vi "Digital Read N Chans.vi"(8 "Error In":errorcluster, 10 "DI Channels":u8[](array[numeric]), 11 "LINX Resource":T1) -> (0 "Error Out":errorcluster, 2 "Values":bool[](array[boolean]), 3 "LINX Resource":T1)   [LabVIEW 2020, in "LMH-LINX.lvlib"]
doc: "Read the values of the specified digital input channels."
uses:
  LMH-LINX.lvlib
  Private/Type Defs/LINX Ref.ctl
  Private/Type Defs/Platform.ctl
  Private/Type Defs/Interface.ctl
  Private/Device/Type Defs/LINX Device Config.ctl
  Private/Device/Type Defs/TCP Config.ctl
  Private/Device/Type Defs/Channels.ctl
  Private/Type Defs/Peripheral.ctl
  Private/Utilties/Generate Error.vi
  Private/Device/Device.lvlib
  Private/Local IO/Local IO.lvlib
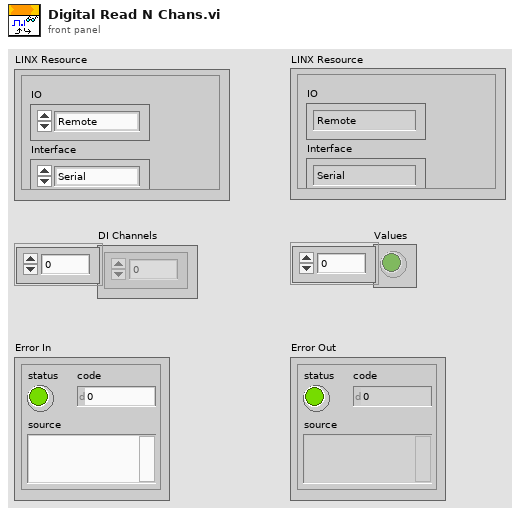
[diagram p1: front panel]
types:
  T1 = typedef "LMH-LINX.lvlib/LINX Ref.ctl" = cluster{"IO":T2, "Interface":T3, "LINX Device Config":T4}
  T2 = typedef "LMH-LINX.lvlib/Platform.ctl" = enum16{"Remote", "Local"}
  T3 = typedef "LMH-LINX.lvlib/Interface.ctl" = enum16{"Serial", "TCP"}
  T4 = typedef "LMH-LINX.lvlib/Device.lvlib/LINX Device Config.ctl" = cluster{"Interface":T3, "COM Port":refnum<visa-resource-name>, "TCP Configuration":T5, "Device Family":u8, "Device ID":u8, "Device Name":string, "TCP Ref":refnum<k5>, "Channels":T6}
  T5 = typedef "LMH-LINX.lvlib/Device.lvlib/TCP Config.ctl" = cluster{"IP Address":string, "Port":u16}
  T6 = typedef "LMH-LINX.lvlib/Channels.ctl" = cluster{"DI":u8[], "DO":u8[], "AI":u8[], "AO":u8[], "PWM":u8[], "QE":u8[], "UART":u8[], "I2C 2":u8[], "SPI":u8[], "CAN":u8[], "Servo":u8[], "AI Ref (V)":dbl, "AI Resolution (Bits)":u8, "AO Ref (V)":dbl, "AO Resolution (Bits)":u8}
  T7 = typedef "LMH-LINX.lvlib/Peripheral.ctl" = enum8{"DI", "DO", "AI", "AO", "PWM", "QE", "UART", "I2C", "SPI", "CAN", "Servo"}
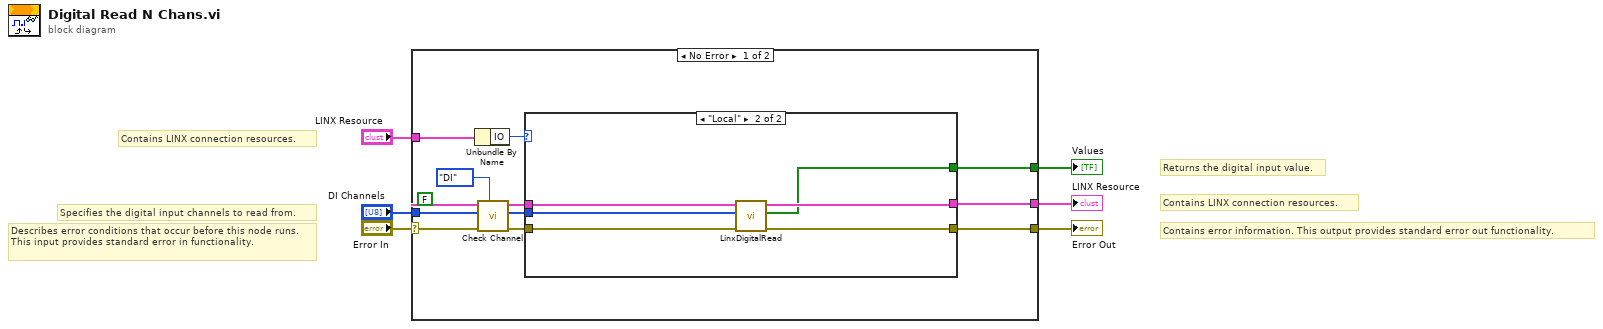
[diagram p0: block diagram]
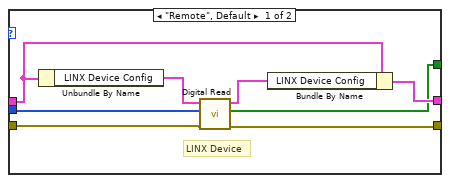
[diagram p2: hidden frame]
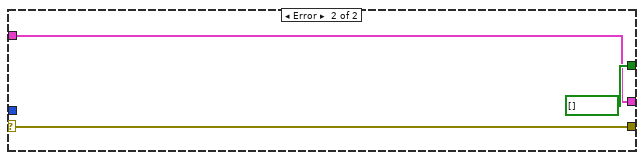
[diagram p3: hidden frame]
diagram:
  # "Specifies the digital input channels to read from."
  # "Returns the digital input value."
  # "Contains LINX connection resources."
  # "Contains error information. This output provides standard error out functionality."
  # "Contains LINX connection resources."
  # "Describes error conditions that occur before this node runs. This input provides standard error in functionality."
  n1 = case shown="No Error" "Error In" {
    selector: "Error In" -> [w8 w34]
    tunnel: [w16 w34] -> w6
    tunnel: [w15 w32] -> w5
    tunnel: [w14 bool[] [] ("Values")] -> w4
    tunnel: "LINX Resource" -> [w10 w32]
    tunnel: "DI Channels" -> [w9 _]
    frame No Error {
      (unwired) FALSE
      n2 = Unbundle By Name(w10) -> ("IO"=w17:T2)
      n3 = call "Check Channel.vi"("Peripheral"=Peripheral."DI", "Error In"=w8, "Channels"=w9, "LINX Resource"=w10) -> ("Error Out"=w13:errorcluster, "Channels"=w12:u8[], "LINX Resource"=w11:T1)  [unwired: 5 in]
      n4 = case shown="\"Local\"" w17 {
        tunnel: w13 -> [w23 w30]
        tunnel: w11 -> [w25 w31]
        tunnel: [w22 w26] -> w16
        tunnel: [w24 w28] -> w15
        tunnel: w12 -> [w19 w29]
        tunnel: [w18 w27] -> w14
        frame "Remote", Default {
          # "LINX Device"
          n5 = Unbundle By Name(w25) -> ("LINX Device Config"=w20:T4)
          n6 = call "Digital Read.vi"("Error In"=w23, "DIO Channels"=w19, "LINX Device Config"=w20) -> ("Error Out"=w22:errorcluster, "Values"=w18:bool[], "LINX Device Config"=w21:T4)  [unwired: 6 in]
          n7 = Bundle By Name(cluster=w25, "LINX Device Config"=w21) -> (w24:T1)
        }
        frame "Local" {
          n8 = call "LinxDigitalRead.vi"("Error In"=w30, "Channels"=w29, "LINX Resource"=w31) -> ("Error Out"=w26:errorcluster, "Values"=w27:bool[], "LINX Resource"=w28:T1)  [unwired: 6 in]
        }
      }
    }
    frame Error {
    }
  }
  "Error Out" <- w6
  "LINX Resource" <- w5
  "Values" <- w4
